vi "Move motor.vi"(6 "Motor params":T1={"Dirección"=enum."Avance", "Tipo"=enum."Simple", "Velocidad (RPM)"=5.0, "Cantidad de pasos"=1, "Avance (mm)"=0.0, "Pasos por rev"=200.0, "Paso del tonillo"=0.0}, 8 "error in":errorcluster, 9 "Acquisition data":T2, 10 "OSC ID mod":i32, 11 "DAQ ID mod":i32) -> (0 "error out":errorcluster)   [LabVIEW 2020, in "GUI.lvlib"]
doc: "Request to move the motor inside the local HL.\n_____\nCreated using DQMH Event Scripter 6.1.0.128."
uses:
  GUI.lvlib
  NI DAQ/Support/Continuous aquisition params.ctl
  NI DAQ/Support/Task list.ctl
  Move motor Argument--cluster.ctl
  NI DAQ/NI DAQ.lvlib
  Support/Motor parameters.ctl
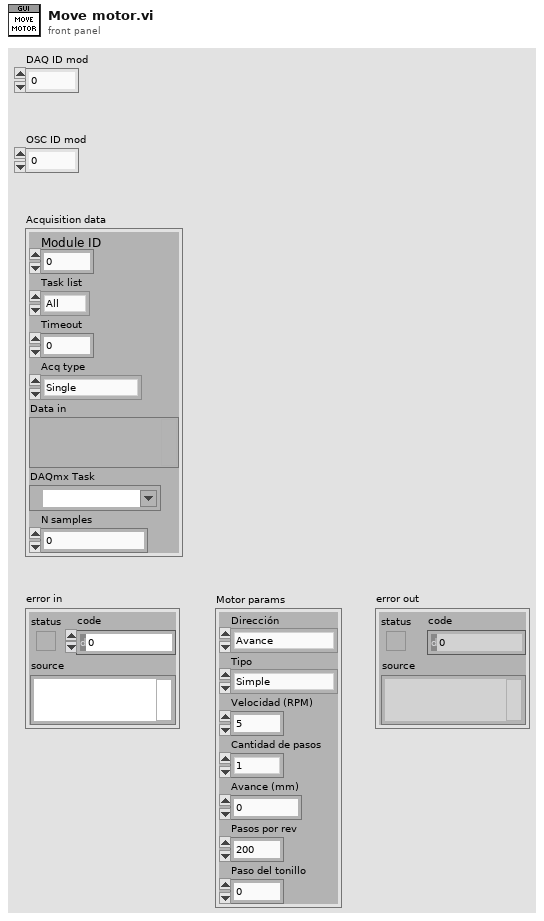
[diagram p1: front panel]
types:
  T1 = typedef "GUI.lvlib/Motor parameters.ctl" = cluster{"Dirección":enum16{"Avance", "Retroceso"}, "Tipo":enum16{"Simple", "Medio paso"}, "Velocidad (RPM)":dbl, "Cantidad de pasos":i32, "Avance (mm)":dbl, "Pasos por rev":dbl, "Paso del tonillo":dbl}
  T2 = typedef "NI DAQ.lvlib/Continuous aquisition params.ctl" = cluster{"Module ID":i32, "Task list":T3, "Timeout":i32, "Acq type":enum16{"Single", "Multiple"}, "Data in":variant, "DAQmx Task":refnum<k21>, "N samples":i32}
  T3 = typedef "NI DAQ.lvlib/Task list.ctl" = enum16{"All", "DO task", "DI task", "AO task", "AI task"}
  T4 = typedef "GUI.lvlib/Move motor Argument--cluster.ctl" = cluster{"Acquisition data":T2, "DAQ ID mod":i32, "OSC ID mod":i32, "Motor params":T1}
  T5 = typedef "GUI.lvlib/Request Events--cluster.ctl" = cluster{"Stop Module":refnum<user-event>, "Show Panel":refnum<user-event>, "Hide Panel":refnum<user-event>, "Get Module Execution Status":refnum<user-event>, "Show Diagram":refnum<user-event>, "Start motor":refnum<user-event>, "Move motor":refnum<user-event>, "Stop motor":refnum<user-event>}
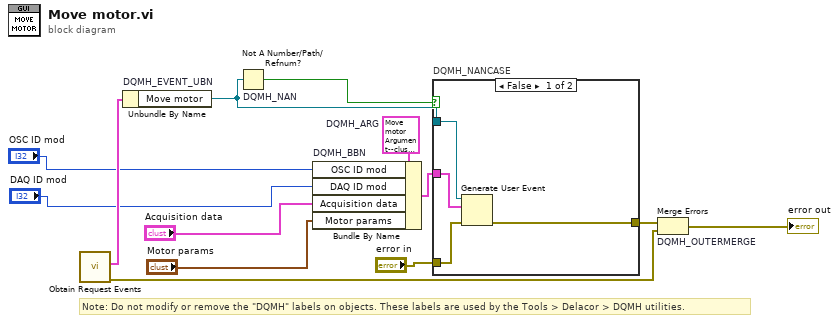
[diagram p0: block diagram]
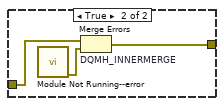
[diagram p2: hidden frame]
diagram:
  w7 = T4 {"Acquisition data"={"Module ID"=0, "Task list"=enum."All", "Timeout"=0, "Acq type"=enum."Single", "Data in"=variant, "DAQmx Task"="", "N samples"=0}, "DAQ ID mod"=0, "OSC ID mod"=0, "Motor params"={"Dirección"=enum."Avance", "Tipo"=enum."Simple", "Velocidad (RPM)"=5.0, "Cantidad de pasos"=1, "Avance (mm)"=0.0, "Pasos por rev"=200.0, "Paso del tonillo"=0.0}}  # DQMH_ARG
  # "Note: Do not modify or remove the \"DQMH\" labels on objects. These labels are used by the Tools > Delacor > DQMH utilities."
  n1 = call "Obtain Request Events.vi"() -> ("error out"=w5:errorcluster, "GUI Request Events"=w4:T5)  [unwired: 10 in]
  n2 = Unbundle By Name "DQMH_EVENT_UBN"(w4) -> ("Move motor"=w9:refnum<user-event>)
  n3 = Not A Number/Path/Refnum? "DQMH_NAN"(number/path/refnum=w9) -> (NaN/Path/Refnum?=w10:bool)
  n4 = Bundle By Name "DQMH_BBN"(cluster=w7, "OSC ID mod"="OSC ID mod", "DAQ ID mod"="DAQ ID mod", "Acquisition data"="Acquisition data", "Motor params"="Motor params") -> (w11:T4)
  n5 = case "DQMH_NANCASE" shown="False" w10 {
    tunnel: "error in" -> [w17 w20]
    tunnel: [w16 w19] -> w8
    tunnel: w9 -> [w15 _]
    tunnel: w11 -> [w14 _]
    frame False {
      n6 = Generate User Event(user event=w15, event data cluster=w14, error in=w17) -> (error out=w16:errorcluster)  [unwired: 1 in, 1 out]
    }
    frame True {
      n7 = call "Module Not Running--error.vi"() -> ("error out"=w18:errorcluster)  [unwired: 11 in]
      n8 = Merge Errors "DQMH_INNERMERGE"(w20, w18) -> (w19:errorcluster)
    }
  }
  n9 = Merge Errors "DQMH_OUTERMERGE"(w8, w5) -> (→"error out":errorcluster)
